vi "Add Step to Tree.vi"(9 "Step Index":i32, 10 "Channels Defined":bool, 11 "Step Settings":T1) -> (1 "Tree Data":T3[](array[typedef]) {"Data Type" items=["Tree Parent"=-1, "Numeric"=0, "String"=1, "Boolean"=2, "Enum"=3]}, 2 "Tree Tags":string[](array[string]), 3 "Tree Items":T2(array[cluster]))   [LabVIEW 2020, in "Sequencer with Output Values.lvlib" / "Sequencer with Output Values.lvclass"]
uses:
  Sequencer with Output Values.lvclass
  Tree Item Settings.ctl
  Data Type.ctl
  Step Settings.ctl
  Global Tree Data.vi
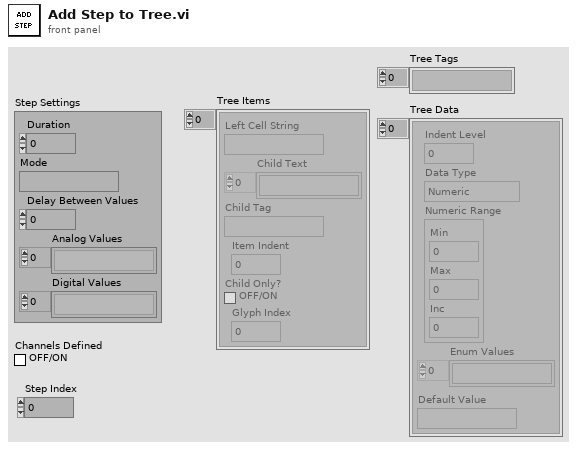
[diagram p1: front panel]
types:
  T1 = typedef "Sequencer with Output Values.lvlib/Sequencer with Output Values.lvclass/Step Settings.ctl" = cluster{"Duration":dbl, "Mode":string, "Delay Between Values":dbl, "Analog Values":string[], "Digital Values":string[]}
  T2 = cluster{"Left Cell String":string, "Child Text":string[], "Child Tag":string, "Item Indent":i32, "Child Only?":bool, "Glyph Index":i32}[]
  T3 = typedef "Sequencer with Output Values.lvlib/Sequencer with Output Values.lvclass/Tree Item Settings.ctl" = cluster{"Indent Level":i32, "Data Type":T4, "Numeric Range":cluster{"Min":dbl, "Max":dbl, "Inc":dbl}, "Enum Values":string[], "Default Value":string}
  T4 = typedef "Sequencer with Output Values.lvlib/Sequencer with Output Values.lvclass/Data Type.ctl" = i16
  T5 = cluster{"Left Cell String":string, "Child Text":string[], "Child Tag":string, "Item Indent":i32, "Child Only?":bool, "Glyph Index":i32}
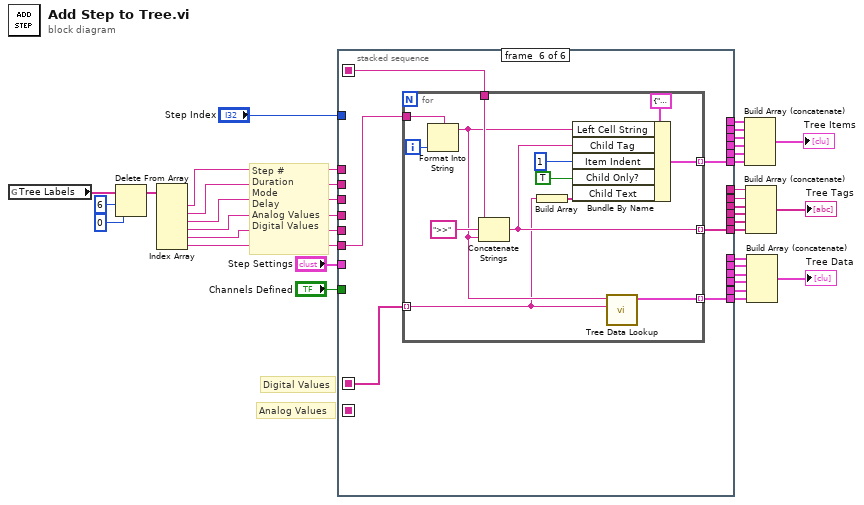
[diagram p0: block diagram]
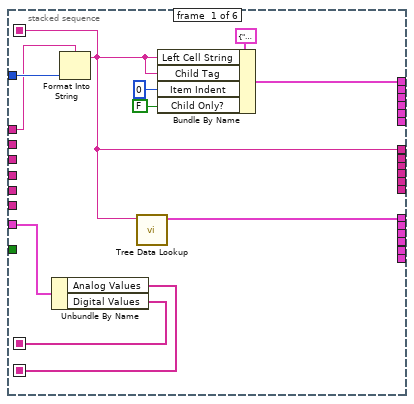
[diagram p2: hidden frame]
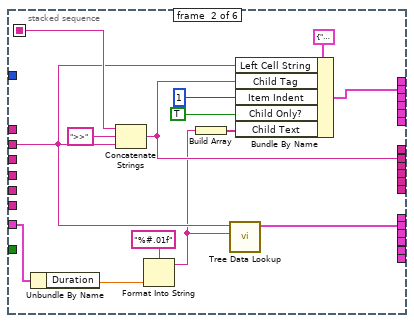
[diagram p3: hidden frame]
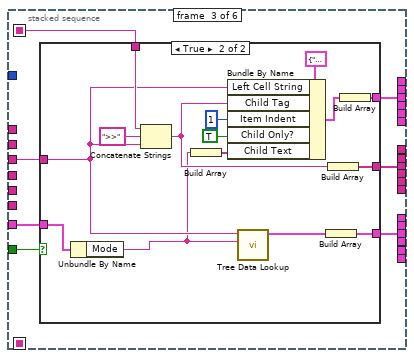
[diagram p4: hidden frame]
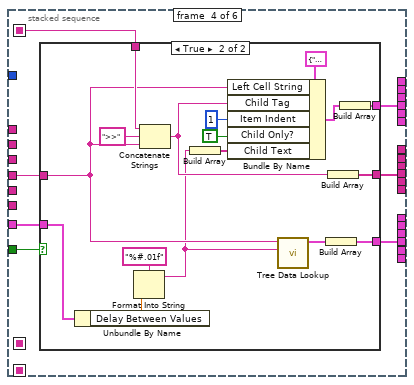
[diagram p6: hidden frame]
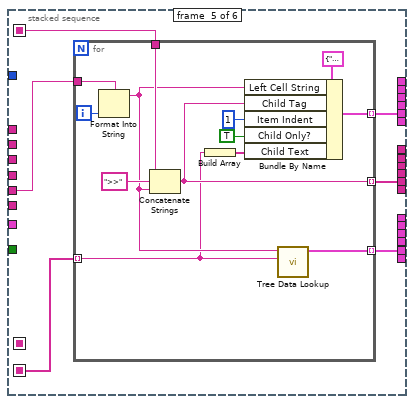
[diagram p8: hidden frame]
diagram:
  # "Analog Values"
  # "Digital Values"
  # "Step #\nDuration\nMode\nDelay\nAnalog Values\nDigital Values"
  n1 = global read "Global Tree Data.vi" "Tree Labels"() -> (w10:string[])
  n2 = Delete From Array(array=w10, length=6, index=0) -> (array with subset deleted=w7:string[])  [unwired: 1 out]
  n3 = Index Array(array=w7) -> (element #1=w6:string, element #2=w2:string, element #3=w3:string, element #4=w4:string, element #5=w5:string, element #6=w1:string)  [unwired: 6 in]
  n4 = stacked-sequence {
    seq-local: [w39 _ _ _ _ _] -> [_ w55 w66 w88 w111 w130]
    seq-local: [w35 _ _ _ _ _] -> [_ _ _ _ _ w129]
    seq-local: [w36 _ _ _ _ _] -> [_ _ _ _ w107 _]
    tunnel: "Step Index" -> [w42 _ _ _ _ _]
    tunnel: w6 -> [w41 _ _ _ _ _]
    tunnel: [w39 _ _ _ _ _] -> w17
    tunnel: [w40 _ _ _ _ _] -> w20
    tunnel: w2 -> [_ w52 _ _ _ _]
    tunnel: [_ w54 _ _ _ _] -> w18
    tunnel: [w38 _ _ _ _ _] -> w13
    tunnel: [_ w53 _ _ _ _] -> w14
    tunnel: "Step Settings" -> [w37 w51 w65 w87 _ _]
    tunnel: [_ w50 _ _ _ _] -> w21
    tunnel: w3 -> [_ _ w64 _ _ _]
    tunnel: [_ _ w63 _ _ _] -> w15
    tunnel: [_ _ w62 _ _ _] -> w19
    tunnel: [_ _ w61 _ _ _] -> w22
    tunnel: w4 -> [_ _ _ w85 _ _]
    tunnel: "Channels Defined" -> [_ _ w60 w86 _ _]
    tunnel: [_ _ _ w84 _ _] -> w26
    tunnel: [_ _ _ w83 _ _] -> w27
    tunnel: [_ _ _ w82 _ _] -> w28
    tunnel: w5 -> [_ _ _ _ w108 _]
    tunnel: [_ _ _ _ w110 _] -> w29
    tunnel: [_ _ _ _ w109 _] -> w30
    tunnel: [_ _ _ _ w106 _] -> w31
    tunnel: [_ _ _ _ _ w128] -> w32
    tunnel: [_ _ _ _ _ w127] -> w33
    tunnel: [_ _ _ _ _ w126] -> w34
    tunnel: w1 -> [_ _ _ _ _ w125]
    frame #0 {
      n5 = Unbundle By Name(w37) -> ("Analog Values"=w36:string[], "Digital Values"=w35:string[])
      n6 = Format Into String(format string=w41, w42) -> (resulting string=w39:string)  [unwired: 2 in, 1 out]
      n7 = call "Tree Data Lookup.vi"("Key"=w39) -> ("Tree Data"=w40:T3)  [unwired: 10 in]
      n8 = Bundle By Name(cluster=T5 {"Left Cell String"="", "Child Text"=[], "Child Tag"="", "Item Indent"=0, "Child Only?"=FALSE, "Glyph Index"=0} ("Item"), "Left Cell String"=w39, "Child Tag"=w39, "Item Indent"=0, "Child Only?"=FALSE) -> (w38:T5)
    }
    frame #1 {
      n9 = Unbundle By Name(w51) -> ("Duration"=w49:dbl)
      n10 = Concatenate Strings(w55, ">>" ("string"), w52) -> (w54:string)
      n11 = Format Into String(format string="%#.01f", w49) -> (resulting string=w47:string)  [unwired: 2 in, 1 out]
      n12 = Build Array(w47) -> (w46:string[])
      n13 = call "Tree Data Lookup.vi"("Value"=w47, "Key"=w52) -> ("Tree Data"=w50:T3)  [unwired: 9 in]
      n14 = Bundle By Name(cluster=T5 {"Left Cell String"="", "Child Text"=[], "Child Tag"="", "Item Indent"=0, "Child Only?"=FALSE, "Glyph Index"=0} ("Item"), "Left Cell String"=w52, "Child Tag"=w54, "Item Indent"=1, "Child Only?"=TRUE, "Child Text"=w46) -> (w53:T5)
    }
    frame #2 {
      n15 = case shown="True" w60 {
        tunnel: w66 -> [_ w77]
        tunnel: w65 -> [_ w76]
        tunnel: w64 -> [_ w75]
        tunnel: [_ w71] -> w63
        tunnel: [_ w70] -> w62
        tunnel: [_ w69] -> w61
        frame False {
          # "If no analog or digital channels configured, no need for mode since this only applies to channels."
        }
        frame True {
          n16 = Unbundle By Name(w76) -> ("Mode"=w68:string)
          n17 = Concatenate Strings(w77, ">>" ("string"), w75) -> (w73:string)
          n18 = Build Array(w68) -> (w67:string[])
          n19 = Bundle By Name(cluster=T5 {"Left Cell String"="", "Child Text"=[], "Child Tag"="", "Item Indent"=0, "Child Only?"=FALSE, "Glyph Index"=0} ("Item"), "Left Cell String"=w75, "Child Tag"=w73, "Item Indent"=1, "Child Only?"=TRUE, "Child Text"=w67) -> (w74:T5)
          n20 = call "Tree Data Lookup.vi"("Value"=w68, "Key"=w75) -> ("Tree Data"=w72:T3)  [unwired: 9 in]
          n21 = Build Array(w72) -> (w69:T3[])
          n22 = Build Array(w73) -> (w70:string[])
          n23 = Build Array(w74) -> (w71:T2)
        }
      }
    }
    frame #3 {
      n24 = case shown="True" w86 {
        tunnel: w88 -> [_ w101]
        tunnel: w87 -> [_ w100]
        tunnel: [_ w96] -> w84
        tunnel: [_ w95] -> w83
        tunnel: [_ w94] -> w82
        tunnel: w85 -> [_ w93]
        frame False {
          # "If no analog or digital channels configured, no need for delay since this only applies to channels."
        }
        frame True {
          n25 = Unbundle By Name(w100) -> ("Delay Between Values"=w91:dbl)
          n26 = Format Into String(format string="%#.01f", w91) -> (resulting string=w89:string)  [unwired: 2 in, 1 out]
          n27 = Concatenate Strings(w101, ">>" ("string"), w93) -> (w98:string)
          n28 = Build Array(w89) -> (w90:string[])
          n29 = Bundle By Name(cluster=T5 {"Left Cell String"="", "Child Text"=[], "Child Tag"="", "Item Indent"=0, "Child Only?"=FALSE, "Glyph Index"=0} ("Item"), "Left Cell String"=w93, "Child Tag"=w98, "Item Indent"=1, "Child Only?"=TRUE, "Child Text"=w90) -> (w99:T5)
          n30 = call "Tree Data Lookup.vi"("Value"=w89, "Key"=w93) -> ("Tree Data"=w97:T3)  [unwired: 9 in]
          n31 = Build Array(w97) -> (w94:T3[])
          n32 = Build Array(w98) -> (w95:string[])
          n33 = Build Array(w99) -> (w96:T2)
        }
      }
    }
    frame #4 {
      n34 = for {
        tunnel: w111 -> [w124]
        tunnel: w108 -> [w119]
        tunnel: [w117] -> w110 mode=indexing
        tunnel: [w116] -> w109 mode=indexing
        tunnel: w107 -> [w112] mode=indexing
        tunnel: [w114] -> w106 mode=indexing
        i -> [w118]
        n35 = Format Into String(format string=w119, w118) -> (resulting string=w115:string)  [unwired: 2 in, 1 out]
        n36 = Concatenate Strings(w124, ">>" ("string"), w115) -> (w116:string)
        n37 = Build Array(w112) -> (w113:string[])
        n38 = Bundle By Name(cluster=T5 {"Left Cell String"="", "Child Text"=[], "Child Tag"="", "Item Indent"=0, "Child Only?"=FALSE, "Glyph Index"=0} ("Item"), "Left Cell String"=w115, "Child Tag"=w116, "Item Indent"=1, "Child Only?"=TRUE, "Child Text"=w113) -> (w117:T5)
        n39 = call "Tree Data Lookup.vi"("Value"=w112, "Key"=w115) -> ("Tree Data"=w114:T3)  [unwired: 9 in]
      }
    }
    frame #5 {
      n40 = for {
        tunnel: w130 -> [w143]
        tunnel: w125 -> [w138]
        tunnel: [w136] -> w126 mode=indexing
        tunnel: [w135] -> w127 mode=indexing
        tunnel: w129 -> [w132] mode=indexing
        tunnel: [w133] -> w128 mode=indexing
        i -> [w137]
        n41 = Format Into String(format string=w138, w137) -> (resulting string=w134:string)  [unwired: 2 in, 1 out]
        n42 = Concatenate Strings(w143, ">>" ("string"), w134) -> (w135:string)
        n43 = Build Array(w132) -> (w131:string[])
        n44 = Bundle By Name(cluster=T5 {"Left Cell String"="", "Child Text"=[], "Child Tag"="", "Item Indent"=0, "Child Only?"=FALSE, "Glyph Index"=0} ("Item"), "Left Cell String"=w134, "Child Tag"=w135, "Item Indent"=1, "Child Only?"=TRUE, "Child Text"=w131) -> (w136:T5)
        n45 = call "Tree Data Lookup.vi"("Value"=w132, "Key"=w134) -> ("Tree Data"=w133:T3)  [unwired: 9 in]
      }
    }
  }
  n46 = Build Array (concatenate)(w13, w14, w15, w26, w29, w34) -> (→"Tree Items":T2)
  n47 = Build Array (concatenate)(w17, w18, w19, w27, w30, w33) -> (→"Tree Tags":string[])
  n48 = Build Array (concatenate)(w20, w21, w22, w28, w31, w32) -> (→"Tree Data":T3[])
